vi "Display Text.vi"(8 "error in (no error)":errorcluster, 10 "Text":string, 11 "Chat Window in":refnum<class "Chat Window.lvclass">) -> (0 "error out":errorcluster, 3 "Chat Window out":refnum<class "Chat Window.lvclass">)   [LabVIEW 2020, in "Chat Window.lvlib" / "Chat Window.lvclass"]
doc: "This VI generates a user event to update the Text to Display indicator in Chat Window:Actor Core."
uses:
  Chat Window.lvclass
  Chat Window.lvclass/Chat Window.ctl
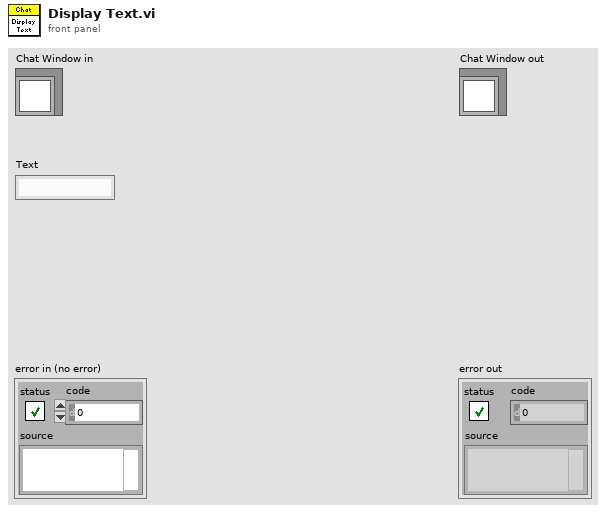
[diagram p1: front panel]
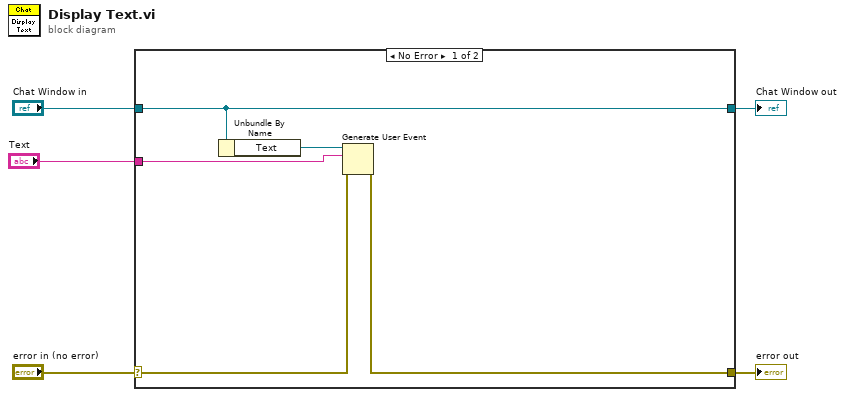
[diagram p0: block diagram]
diagram:
  n1 = case shown="No Error" "error in (no error)" {
    selector: "error in (no error)" -> [w7 w12]
    tunnel: [w6 w12] -> w4
    tunnel: [w10 w11] -> w2
    tunnel: "Chat Window in" -> [w10 w11]
    tunnel: "Text" -> [w8 _]
    frame No Error {
      n2 = Unbundle By Name(w10) -> ("Text"=w9:refnum<user-event>)
      n3 = Generate User Event(user event=w9, event data cluster=w8, error in=w7) -> (error out=w6:errorcluster)  [unwired: 1 in, 1 out]
    }
    frame Error {
    }
  }
  "error out" <- w4
  "Chat Window out" <- w2
